vi "StahlPS_USB.constructor.vi"(0 "name":string, 2 "data in":string, 5 "error in(no error)":errorcluster) -> (14 "i ref out":refnum<vi>, 16 "data out":string, 19 "error out":errorcluster)   [LabVIEW 2014, in "StahlPS_USB.lvlib"]
doc: "This is the constructor of a class.\n\nLicense Agreement for this software:\n\nCopyright (C)\nGesellschaft für Schwerionenforschung, GSI\nPlanckstr. 1\n64291 Darmstadt\nGermany\n\nContact: D.Beck@gsi.de \n\nThis program is free software; you can redistribute it and/or modify it under the terms of the \nGNU General Public License as published by the Free Software Foundation; either version 2 of \nthe license, or (at your option) any later version.\n\nThis program is distributed in the hope that it will be useful, but WITHOUT ANY WARRANTY; \nwithout even the implied warranty of MERCHANTABILITY or FITNESS FOR A PARTICULAR PURPOSE. See the GNU General License for more details (http://www.gnu.org).\n\nGesellschaft für Schwerionenforschung, GSI\nPlanckstr. 1, 64291 Darmstadt, Germany\nFor all questions and ideas contact: M.Richter@gsi.de, H.Brand@gsi.de or D.Beck@gsi.de.\nLast update: 16-JUN-2004"
uses:
  StahlPS_USB.lvlib
  CSCore/CSApplicationBaseClasses/DeviceBase/DeviceBase.myEventNames.ctl
  CSCore/CSApplicationBaseClasses/PSChannelBase/PSChannelBase.myEventNames.ctl
  CSlibraries/UtilityLib/UtilityLib.valueStatus.ctl
  CSCore/CSSystem/CSSystemLib/CSSystemLib.lvlib
  CSCore/CSApplicationBaseClasses/PSChannelBase/PSChannelBase.lvlib
  CSCore/CSApplicationBaseClasses/DeviceBase/DeviceBase.lvlib
  CSlibraries/UtilityLib/UtilityLib.lvlib
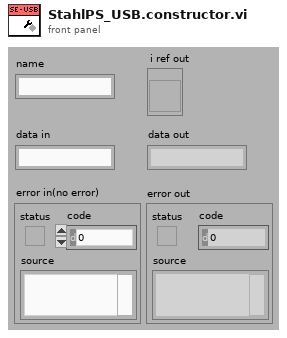
[diagram p1: front panel]
types:
  T1 = typedef "UtilityLib.lvlib/UtilityLib.valueStatus.ctl" = enum16{"no info available", "stand by/off", "on", "warning", "alarm/malfunction", "not implemented", "user action required", "important information", "system default", "control default", "indicator default", "button default"}
  T2 = enum16{"SetAttribute", "GetAttribute", "CreateAttribute", "DestroyAttribute", "DestroyAllAtributes"}
  T3 = typedef "PSChannelBase.lvlib/PSChannelBase.myEventNames.ctl" = enum16{"lvmsg://EmergencyOff", "lvmsg://SetOnOff", "lvmsg://GetOnOff", "lvmsg://SetVoltage", "lvmsg://GetVoltage", "lvmsg://SetCurrent", "lvmsg://GetCurrent", "lvmsg://SetTripCurrent", "lvmsg://GetTripCurrent", "lvmsg://SetRampUpSpeed", "lvmsg://GetRampUpSpeed", "lvmsg://SetRampDownSpeed", "lvmsg://GetRampDownSpeed", "lvmsg://SetChannelOnOff", "lvmsg://GetChannelOnOff", "lvmsg://SetChannelVoltage", "lvmsg://GetChannelVoltage", "lvmsg://SetChannelCurrent", "lvmsg://GetChannelCurrent", "lvmsg://SetChannelTripCurrent", "lvmsg://GetChannelTripCurrent", "lvmsg://SetChannelRampUpSpeed", "lvmsg://GetChannelRampUpSpeed", "lvmsg://SetChannelRampDownSpeed", "lvmsg://GetChannelRampDownSpeed"}
  T4 = typedef "DeviceBase.lvlib/DeviceBase.myEventNames.ctl" = enum16{"lvmsg://Initialize", "lvmsg://Close", "lvmsg://Configure", "lvmsg://Reset", "lvmsg://IDQuery"}
  T5 = typedef "StahlPS_USB.lvlib/StahlPS_USB.i attribute.ctl" = cluster{"VISA resource name":refnum<visa-resource-name>, "Type":string, "MaxVoltage":dbl, "MinVoltage":dbl, "Elektrode Names":string[]}
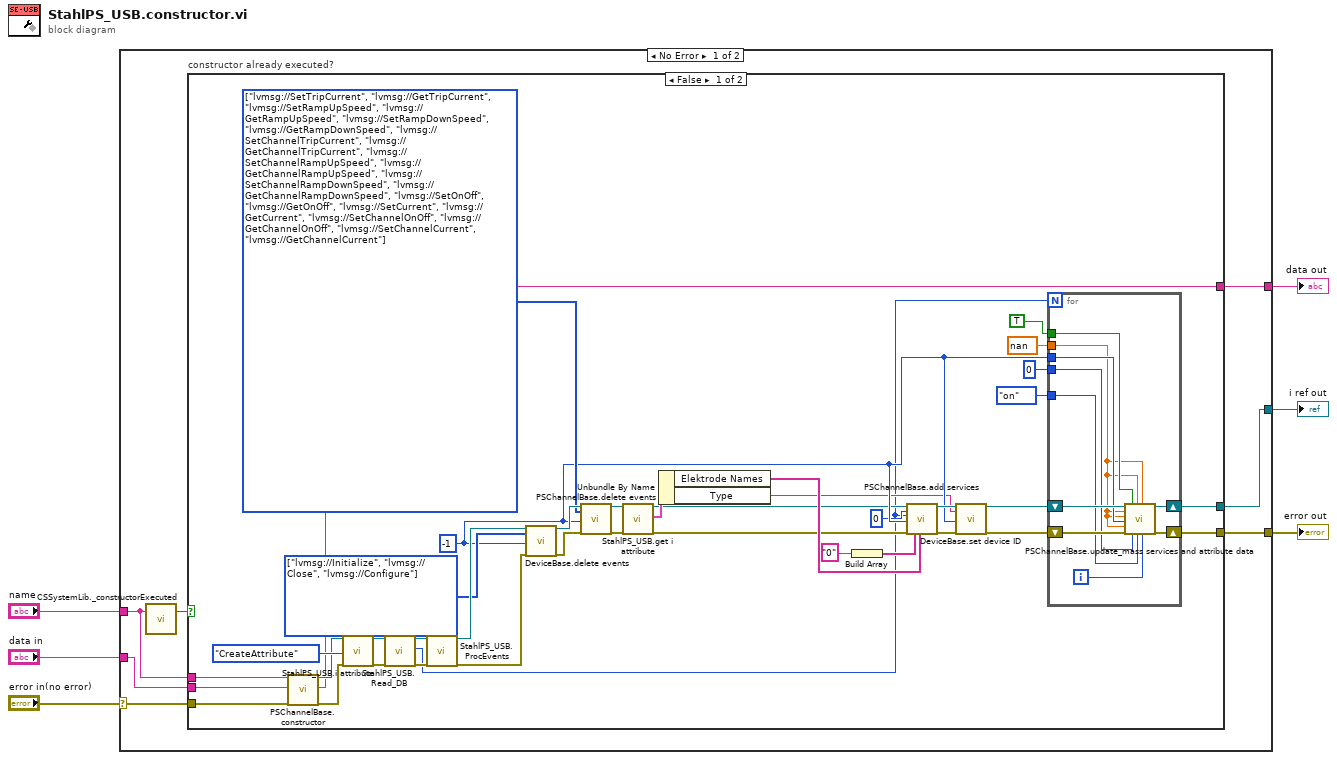
[diagram p0: block diagram]
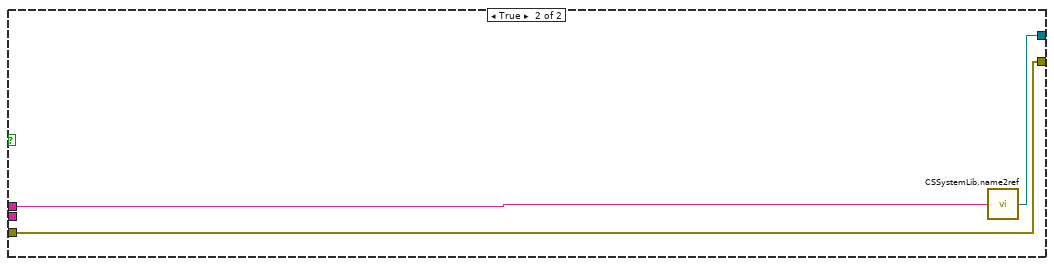
[diagram p2: hidden frame]
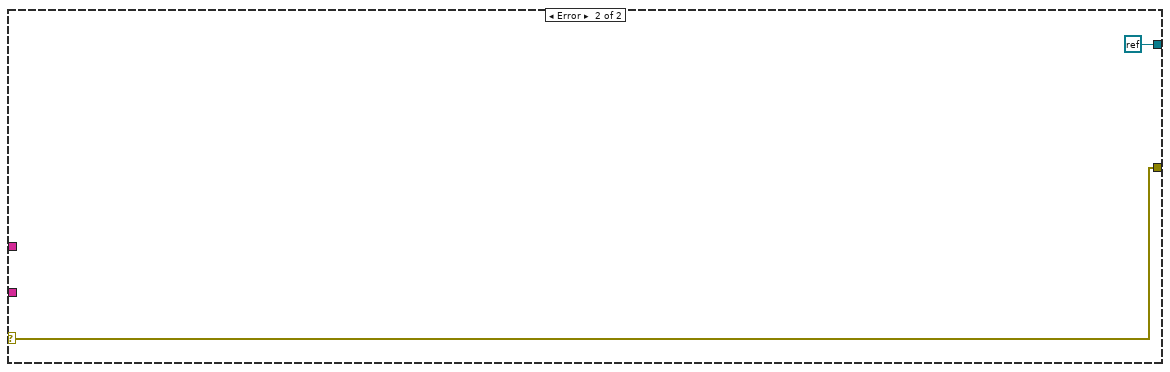
[diagram p3: hidden frame]
diagram:
  n1 = case shown="No Error" "error in(no error)" {
    selector: "error in(no error)" -> [w11 w66]
    tunnel: "name" -> [w10 _]
    tunnel: [w13 refnum<k0> refnum] -> w5
    tunnel: [w12 w66] -> w4
    tunnel: "data in" -> [w8 _]
    tunnel: [w7 _] -> w1
    frame No Error {
      n2 = call "CSSystemLib._constructorExecuted.vi"("name"=w10) -> ("constructor executed?"=w9:bool)  [unwired: 18 in]
      n3 = case "constructor already executed?" shown="False" w9 {
        tunnel: [w30 w64] -> w13
        tunnel: [w31 w63] -> w12
        tunnel: w11 -> [w52 w63]
        tunnel: w10 -> [w21 w65]
        tunnel: w8 -> [w51 _]
        tunnel: [w45 _] -> w7
        frame False {
          w37 = T3[] [enum."lvmsg://SetTripCurrent", enum."lvmsg://GetTripCurrent", enum."lvmsg://SetRampUpSpeed", enum."lvmsg://GetRampUpSpeed", enum."lvmsg://SetRampDownSpeed", enum."lvmsg://GetRampDownSpeed", enum."lvmsg://SetChannelTripCurrent", enum."lvmsg://GetChannelTripCurrent", enum."lvmsg://SetChannelRampUpSpeed", enum."lvmsg://GetChannelRampUpSpeed", enum."lvmsg://SetChannelRampDownSpeed", enum."lvmsg://GetChannelRampDownSpeed", enum."lvmsg://SetOnOff", enum."lvmsg://GetOnOff", enum."lvmsg://SetCurrent", enum."lvmsg://GetCurrent", enum."lvmsg://SetChannelOnOff", enum."lvmsg://GetChannelOnOff", enum."lvmsg://SetChannelCurrent", enum."lvmsg://GetChannelCurrent"] items=["lvmsg://EmergencyOff", "lvmsg://SetOnOff", "lvmsg://GetOnOff", "lvmsg://SetVoltage", "lvmsg://GetVoltage", "lvmsg://SetCurrent", "lvmsg://GetCurrent", "lvmsg://SetTripCurrent", "lvmsg://GetTripCurrent", "lvmsg://SetRampUpSpeed", "lvmsg://GetRampUpSpeed", "lvmsg://SetRampDownSpeed", "lvmsg://GetRampDownSpeed", "lvmsg://SetChannelOnOff", "lvmsg://GetChannelOnOff", "lvmsg://SetChannelVoltage", "lvmsg://GetChannelVoltage", "lvmsg://SetChannelCurrent", "lvmsg://GetChannelCurrent", "lvmsg://SetChannelTripCurrent", "lvmsg://GetChannelTripCurrent", "lvmsg://SetChannelRampUpSpeed", "lvmsg://GetChannelRampUpSpeed", "lvmsg://SetChannelRampDownSpeed", "lvmsg://GetChannelRampDownSpeed"] ("events")
          w40 = T4[] [enum."lvmsg://Initialize", enum."lvmsg://Close", enum."lvmsg://Configure"] items=["lvmsg://Initialize", "lvmsg://Close", "lvmsg://Configure", "lvmsg://Reset", "lvmsg://IDQuery"] ("events")
          w20 = -1 ("ms timeout (10000)")
          n4 = call "PSChannelBase.constructor.vi"("name"=w21, "data in"=w51, "error in (no error)"=w52) -> ("i ref out"=w46:refnum<vi>, "data out"=w45:string, "error out"=w47:errorcluster)  [unwired: 14 in]
          n5 = call "StahlPS_USB.i attribute.vi"("VI Refnum"=w46, "Action"=T2."CreateAttribute", "error in (no error)"=w47) -> ("VI Refnum out"=w49:refnum<vi>, "error out"=w48:errorcluster)  [unwired: 14 in, 1 out]
          n6 = call "StahlPS_USB.Read_DB.vi"("i ref in"=w49, "error in (no error)"=w48) -> ("i ref out"=w44:refnum<vi>, "NofChannels"=w14:i32, "error out (no error)"=w43:errorcluster)  [unwired: 15 in]
          n7 = call "StahlPS_USB.ProcEvents.vi"("i ref in"=w44, "error in"=w43) -> ("i ref out"=w42:refnum<vi>, "error out"=w41:errorcluster)  [unwired: 16 in]
          n8 = call "DeviceBase.delete events.vi"("i ref in"=w42, "events"=w40, "ms timeout (10000)"=w20, "error in (no error)"=w41) -> ("i ref out"=w39:refnum<vi>, "error out"=w38:errorcluster)  [unwired: 13 in, 1 out]
          n9 = call "PSChannelBase.delete events.vi"("i ref in"=w39, "events"=w37, "ms timeout (10000)"=w20, "error in (no error)"=w38) -> ("i ref out"=w35:refnum<vi>, "error out"=w36:errorcluster)  [unwired: 13 in, 1 out]
          n10 = call "StahlPS_USB.get i attribute.vi"("i ref in"=w35, "error in (no error)"=w36) -> ("i ref out"=w17:refnum<vi>, "i attribute"=w34:T5, "error out"=w16:errorcluster)  [unwired: 15 in]
          n11 = Unbundle By Name(w34) -> ("Elektrode Names"=w19:string[], "Type"=w18:string)
          n12 = Build Array("0") -> (w32:string[])
          n13 = call "PSChannelBase.add services.vi"("i ref in"=w17, "defaultChannelIndex"=0, "nofChannels"=w14, "ms timeout (10000)"=w20, "error in (no error)"=w16, "physicalNames"=w32, "logicalNames"=w19) -> ("i ref out"=w26:refnum<vi>, "error out"=w24:errorcluster)  [unwired: 10 in, 1 out]
          n14 = call "DeviceBase.set device ID.vi"("i ref in"=w26, "deviceID"=w18, "ms timeout (10000)"=w20, "error in (no error)"=w24) -> ("i ref out"=w25:refnum<vi>, "error out"=w23:errorcluster)  [unwired: 13 in, 1 out]
          n15 = for {
            N: w14 -> [_]
            shift-right: [w60] -> w31
            shift-left: w23 -> [w61]
            shift-right: [w58] -> w30
            shift-left: w25 -> [w59]
            tunnel: UtilityLib.valueStatus."on" ("valueStatus") -> [w57]
            tunnel: nan -> [w54]
            tunnel: w20 -> [w56]
            tunnel: TRUE -> [w55]
            tunnel: 0 -> [w53]
            i -> [w62]
            n16 = call "PSChannelBase.update_mass services and attribute data.vi"("i ref in"=w59, "tripCurrent"=w54, "rampUpSpeed"=w54, "ms timeout (10000)"=w56, "rampDownSpeed"=w54, "error in (no error)"=w61, "onOff"=w55, "status"=w53, "voltage"=w54, "valueStatus"=w57, "current"=w54, "channelNumber"=w62) -> ("i ref out"=w58:refnum<vi>, "error out"=w60:errorcluster)  [unwired: 5 in, 1 out]
          }
        }
        frame True {
          n17 = call "CSSystemLib.name2ref.vi"("name"=w65) -> ("obj refnum"=w64:refnum<vi>)
        }
      }
    }
    frame Error {
    }
  }
  "i ref out" <- w5
  "error out" <- w4
  "data out" <- w1
